vi "SVT UFF58 Write Records 1 to 3.vi"(0 "function refnum":refnum<k20>, 5 "ID lines (1-3)":T1, 11 "error in (no error)":errorcluster) -> (4 "dup function refnum":refnum<k20>, 15 "error out":errorcluster)   [LabVIEW 2017, in "SoundVib_UFF58.lvlib"]
doc: "Writes the values of records 1, 2, and 3 of the UFF58 (universal file format) file. Record 1 typically is used for the function description. Record 3 typically is used to identify when the function was created."
uses:
  <vilib>/addons/Sound and Vibration/svt_UFF58/SoundVib_UFF58.lvlib
  <vilib>/addons/Sound and Vibration/svt_UFF58/subVIs/sv_IDLines123.ctl
  <vilib>/Platform/storage/Storage.llb/Set Property (String).vi
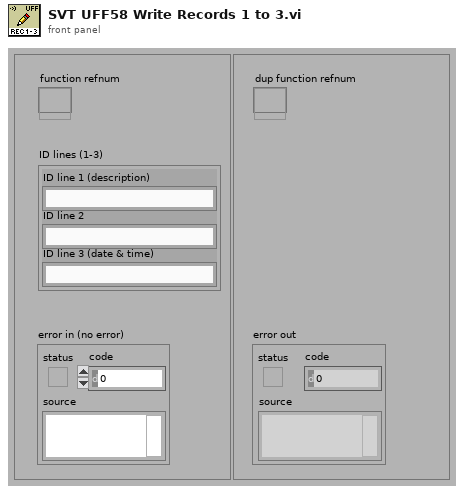
[diagram p1: front panel]
types:
  T1 = typedef "SoundVib_UFF58.lvlib/sv_IDLines123.ctl" = cluster{"ID line 1 (description)":string, "ID line 2":string, "ID line 3 (date & time)":string}
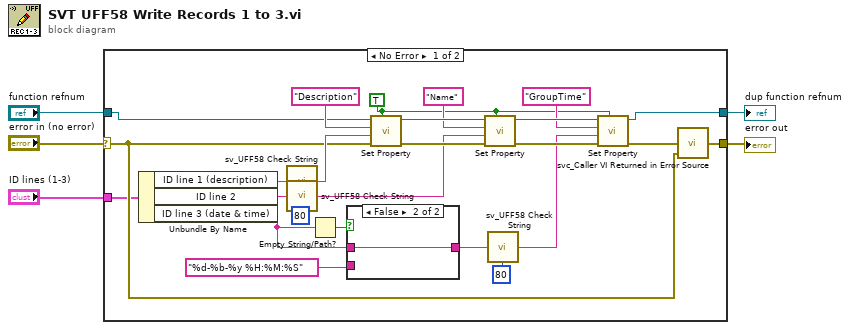
[diagram p0: block diagram]
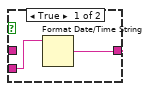
[diagram p2: hidden frame]
diagram:
  n1 = case shown="No Error" "error in (no error)" {
    selector: "error in (no error)" -> [w8 w34]
    tunnel: "function refnum" -> [w29 w35]
    tunnel: "ID lines (1-3)" -> [w7 _]
    tunnel: [w15 w35] -> w1
    tunnel: [w9 w34] -> w4
    frame No Error {
      w6 = TRUE ("Create if not found (no:F)")
      w14 = 80 ("length (rest)")
      n2 = Unbundle By Name(w7) -> ("ID line 1 (description)"=w23:string, "ID line 2"=w22:string, "ID line 3 (date & time)"=w17:string)
      n3 = call <vilib>:"sv_UFF58 Check String.vi"("field value"=w23, "field length"=w14) -> ("output string"=w21:string)  [unwired: 12 in, 1 out]
      n4 = call <vilib>:"sv_UFF58 Check String.vi"("field value"=w22, "field length"=w14) -> ("output string"=w20:string)  [unwired: 12 in, 1 out]
      n5 = Empty String/Path?(string/path=w17) -> (empty?=w16:bool)
      n6 = case shown="False" w16 {
        tunnel: [w32 w33] -> w12
        tunnel: w17 -> [_ w33]
        tunnel: "%d-%b-%y %H:%M:%S" ("time format string (%c)") -> [w31 _]
        frame True {
          n7 = Format Date/Time String(time format string (%c)=w31) -> (date/time string=w32:string)  [unwired: 2 in]
        }
        frame False {
        }
      }
      n8 = call-poly <vilib>:"Set Property.vi"("Create if not found (no:F)"=w6, "error in (no error)"=w8, "Value"=w21, "Property name"="Description", "storage refnum"=w29) -> ("error out"=w26:errorcluster, "storage refnum out"=w28:refnum<k20>)  [unwired: 5 in]
      n9 = call-poly <vilib>:"Set Property.vi"("Create if not found (no:F)"=w6, "error in (no error)"=w26, "Value"=w20, "Property name"="Name", "storage refnum"=w28) -> ("error out"=w24:errorcluster, "storage refnum out"=w25:refnum<k20>)  [unwired: 5 in]
      n10 = call <vilib>:"sv_UFF58 Check String.vi"("field value"=w12, "field length"=80 ("length (rest)")) -> ("output string"=w13:string)  [unwired: 12 in, 1 out]
      n11 = call-poly <vilib>:"Set Property.vi"("Create if not found (no:F)"=w6, "error in (no error)"=w24, "Value"=w13, "Property name"="GroupTime", "storage refnum"=w25) -> ("error out"=w10:errorcluster, "storage refnum out"=w15:refnum<k20>)  [unwired: 5 in]
      n12 = call <vilib>:"svc_Caller VI Returned in Error Source.vi"("warning input to caller"=w8, "error in (no error)"=w10) -> ("error out"=w9:errorcluster)  [unwired: 3 in]
    }
    frame Error {
    }
  }
  "error out" <- w4
  "dup function refnum" <- w1
